vi "2 Antenna WB Spectrum Sense (Averaged).vi"() -> ()   [LabVIEW 2011]
panel:
  out "FFT Power Spectrum Rx2":cluster{"f0":dbl, "df":dbl, "IQ":dbl[]}(graph)={"f0"=87750000.0, "df"=1000.0, "IQ"=array[20500 elements]}
  in  "Averaging Parameters":T1={"averaging mode"=enum."RMS averaging", "weighting mode"=enum."Linear", "number of averages"=10} {"number of averages" min=1}
  in  "stop":bool
  in  "Rx Parameters":T2={"IQ Sampling\nRate [S/sec]"=1000000.0, "Acq Duration [sec]"=0.001, "Start Carrier [Hz]"=88000000.0, "Stop Carrier [Hz]"=108000000.0, "Gain [dB]"=25.0, "Active Antenna"="RX2", "Reference Source"="Internal", "Timebase Source"="Internal"} {"Gain [dB]" format="%#_4g"; "Stop Carrier [Hz]" min=50000000.0 max=6000000000.0 step=1000.0 format="%#.15p"; "Start Carrier [Hz]" min=50000000.0 max=6000000000.0 step=1000.0 format="%#.15p"; "Acq Duration [sec]" min=0.0 step=0.001 format="%#.6p"; "IQ Sampling\nRate [S/sec]" format="%#_6p"}
  in  "Display Settings":cluster{"display unit":u16, "log/linear":u16}={"display unit"=2, "log/linear"=2} {"log/linear" items=["Linear", "dB", "dBm"]; "display unit" items=["Vrms", "Vpk", "Vrms^2", "Vpk^2", "Vrms/rtHz", "Vpk/rtHz", "Vrms^2/Hz", "Vpk^2/Hz"]}
  out "error out":errorcluster
  out "FFT Power Spectrum Rx1":cluster{"f0":dbl, "df":dbl, "IQ":dbl[]}(graph)={"f0"=87750000.0, "df"=1000.0, "IQ"=array[20500 elements]}
  in  "USRP IP Address":refnum<k15>="192.168.12.4"
  # "Wideband Spectrum (Averaged)"
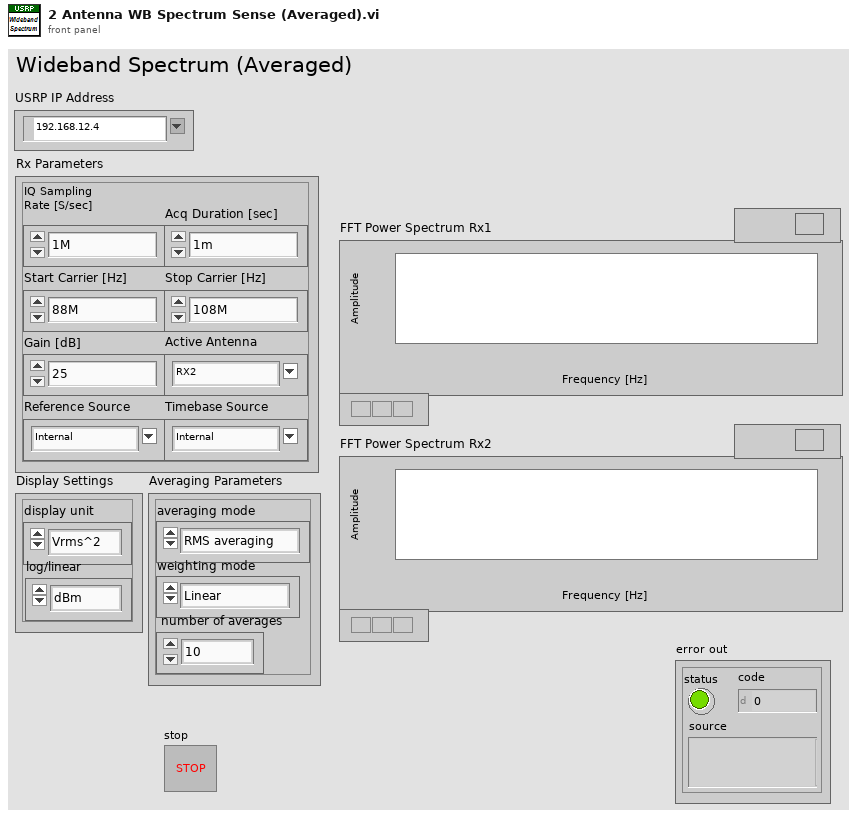
[diagram p1: front panel]
types:
  T1 = cluster{"averaging mode":enum16{"No averaging", "Vector averaging", "RMS averaging", "Peak hold"}, "weighting mode":enum16{"Linear", "Exponential"}, "number of averages":u32}
  T2 = cluster{"IQ Sampling\nRate [S/sec]":dbl, "Acq Duration [sec]":dbl, "Start Carrier [Hz]":dbl, "Stop Carrier [Hz]":dbl, "Gain [dB]":dbl, "Active Antenna":string, "Reference Source":string, "Timebase Source":string}
  T3 = typedef "subFrameParams.ctl" = cluster{"IQ Rate":dbl, "Frames":i32, "Length of Subset":i32, "Start Index of Subset":i32, "Start Carrier [Hz]":dbl, "Stop Carrier [Hz]":dbl, "Acq Duration [sec]":dbl}
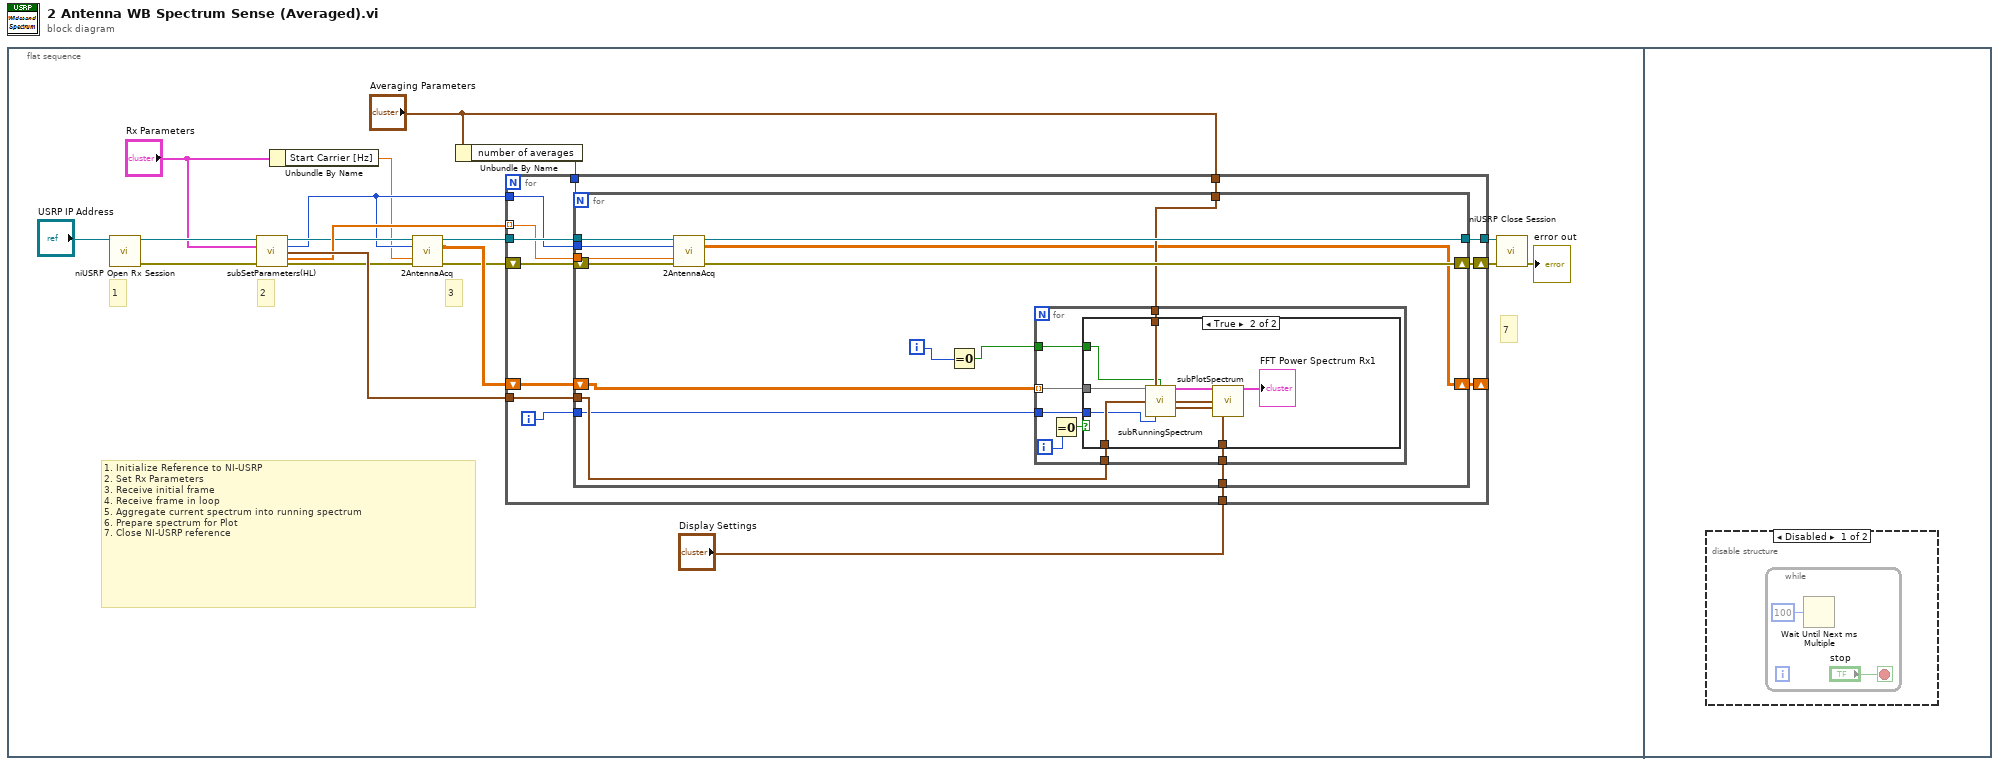
[diagram p0: block diagram]
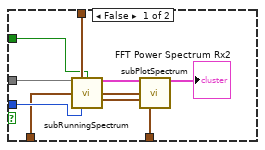
[diagram p2: hidden frame]
diagram:
  n1 = flat-sequence {
    frame #0 {
      # "7"
      # "3"
      # "2"
      # "1"
      # "1. Initialize Reference to NI-USRP\n2. Set Rx Parameters\n3. Receive initial frame\n4. Receive frame in loop\n5. Aggregate current spectrum into running spectrum\n6. Prepare spectrum for Plot\n7. Close NI-USRP reference"
      n2 = call <instrlib>:"niUSRP Open Rx Session.vi"("device names"="USRP IP Address") -> ("session handle out"=w15:refnum<k15>, "error out"=w14:errorcluster)  [unwired: 13 in]
      n3 = call "subSetParameters(HL).vi"("IVI Refnum in"=w15, "Rx Parameters"="Rx Parameters", "error in (no error)"=w14) -> ("IVI Refnum out"=w7:refnum<k15>, "samples per acquisition"=w6:i32, "Frame Parameters"=w12:T3, "test carrier frequencies"=w11:dbl[], "error out"=w5:errorcluster)  [unwired: 8 in]
      n4 = Unbundle By Name("Rx Parameters") -> ("Start Carrier [Hz]"=w4:dbl)
      n5 = call "2AntennaAcq.vi"("IVI Refnum in"=w7, "samples per acquisition"=w6, "Carrier"=w4, "error in (no error)"=w5) -> ("IVI Refnum out"=w3:refnum<k15>, "data"=w2:cdb[][], "error out"=w1:errorcluster)  [unwired: 9 in]
      n6 = Unbundle By Name("Averaging Parameters") -> ("number of averages"=w9:u32)
      n7 = for {
        tunnel: w3 -> [w32]
        tunnel: w6 -> [w25]
        tunnel: [w31] -> w18
        shift-right: [w24] -> w17
        shift-left: w1 -> [w30]
        shift-right: [w23] -> _
        shift-left: w2 -> [w29]
        tunnel: w12 -> [w28]
        tunnel: w11 -> [w27] mode=indexing
        tunnel: "Display Settings" -> [w26]
        tunnel: w9 -> [w22]
        tunnel: "Averaging Parameters" -> [w21]
        i -> [w20]
        n8 = for {
          N: w22 -> [_]
          tunnel: w32 -> [w46]
          tunnel: [w45] -> w31
          tunnel: w28 -> [w38]
          tunnel: w27 -> [w43]
          tunnel: w26 -> [w40]
          tunnel: w25 -> [w42]
          shift-right: [w36] -> w23
          shift-left: w29 -> [w37]
          shift-right: [w41] -> w24
          shift-left: w30 -> [w44]
          tunnel: w21 -> [w39]
          tunnel: w20 -> [w35]
          i -> [w34]
          n9 = call "2AntennaAcq.vi"("IVI Refnum in"=w46, "samples per acquisition"=w42, "Carrier"=w43, "error in (no error)"=w44) -> ("IVI Refnum out"=w45:refnum<k15>, "data"=w36:cdb[][], "error out"=w41:errorcluster)  [unwired: 9 in]
          n10 = Equal To 0?(x=w34) -> (x = 0?=w33:bool)
          n11 = for {
            tunnel: w40 -> [w54]
            tunnel: w39 -> [w51]
            tunnel: w38 -> [w50]
            tunnel: w37 -> [w49] mode=indexing
            tunnel: w33 -> [w48]
            tunnel: w35 -> [w47]
            i -> [w52]
            n12 = Equal To 0?(x=w52) -> (x = 0?=w53:bool)
            n13 = case shown="True" w53 {
              tunnel: w54 -> [w56 w70]
              tunnel: w49 -> [w59 w69]
              tunnel: w51 -> [w58 w68]
              tunnel: w50 -> [w57 w67]
              tunnel: w48 -> [w55 w65]
              tunnel: w47 -> [w60 w66]
              frame False {
                n14 = call "subRunningSpectrum.vi"("Input Baseband IQ"=w59, "averaging parameters"=w58, "restart averaging (T)"=w55, "Frame Parameters"=w57, "Iteration"=w60) -> ("Spectrum to Plot"=w64:cluster{"f0":dbl, "df":dbl, "IQ":dbl[]}, "Frame Parameters out"=w63:T3, "window properties"=w62:cluster{"eq noise BW":dbl, "coherent gain":dbl})  [unwired: 7 in, 1 out]
                n15 = call "subPlotSpectrum.vi"("Spectrum to Plot"=w64, "Frame Parameters"=w63, "window properties"=w62, "Display"=w56) -> ("Spectrum to Plot"=→"FFT Power Spectrum Rx2":cluster{"f0":dbl, "df":dbl, "IQ":dbl[]})  [unwired: 11 in]
              }
              frame True {
                n16 = call "subRunningSpectrum.vi"("Input Baseband IQ"=w69, "averaging parameters"=w68, "restart averaging (T)"=w65, "Frame Parameters"=w67, "Iteration"=w66) -> ("Spectrum to Plot"=w74:cluster{"f0":dbl, "df":dbl, "IQ":dbl[]}, "Frame Parameters out"=w73:T3, "window properties"=w72:cluster{"eq noise BW":dbl, "coherent gain":dbl})  [unwired: 7 in, 1 out]
                n17 = call "subPlotSpectrum.vi"("Spectrum to Plot"=w74, "Frame Parameters"=w73, "window properties"=w72, "Display"=w70) -> ("Spectrum to Plot"=→"FFT Power Spectrum Rx1":cluster{"f0":dbl, "df":dbl, "IQ":dbl[]})  [unwired: 11 in]
              }
            }
          }
        }
      }
      n18 = call <instrlib>:"niUSRP Close Session.vi"("session handle"=w18, "error in (no error)"=w17) -> ("error out"=→"error out":errorcluster)  [unwired: 13 in]
    }
    frame #1 {
      n19 = disable-structure shown="Disabled" {
        frame Disabled {
          n20 = while {
            stop <- "stop" stop-if-true
            n21 = Wait Until Next ms Multiple(millisecond multiple=u32 100) -> ()  [unwired: 1 out]
          }
        }
        frame Enabled {
        }
      }
    }
  }
